vi "SubVi_Flancos.vi"(11 "Alarmas":bool[](array[boolean])) -> (0 "Conteo 3":bool, 1 "Conteo 2":bool, 2 "Conteo 1":bool, 3 "Conteo":bool)   [LabVIEW 2017]
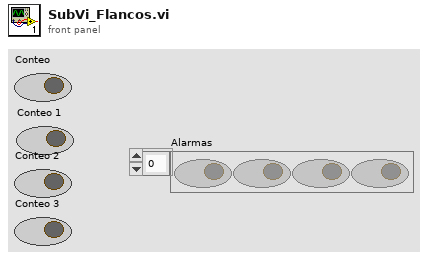
[diagram p1: front panel]
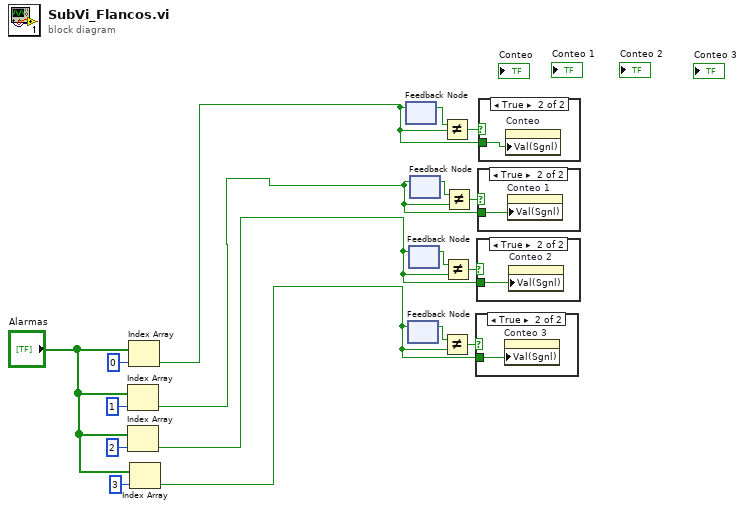
[diagram p0: block diagram]
diagram:
  n1 = Index Array(array="Alarmas", index=1) -> (element=w2:bool)
  n2 = Index Array(array="Alarmas", index=2) -> (element=w3:bool)
  n3 = Index Array(array="Alarmas", index=0) -> (element=w1:bool)
  n4 = Index Array(array="Alarmas", index=3) -> (element=w4:bool)
  n5 = feedback #1() -> (w17:bool)  [unwired: 1 in]
  n6 = feedback-in #1(w1) -> ()
  n7 = feedback #2() -> (w11:bool)  [unwired: 1 in]
  n8 = feedback-in #2(w4) -> ()
  n9 = feedback #3() -> (w13:bool)  [unwired: 1 in]
  n10 = feedback-in #3(w3) -> ()
  n11 = feedback #4() -> (w15:bool)  [unwired: 1 in]
  n12 = feedback-in #4(w2) -> ()
  n13 = Not Equal?(x=w17, y=w1) -> (x != y?=w16:bool)
  n14 = Not Equal?(x=w11, y=w4) -> (x != y?=w10:bool)
  n15 = Not Equal?(x=w13, y=w3) -> (x != y?=w12:bool)
  n16 = Not Equal?(x=w15, y=w2) -> (x != y?=w14:bool)
  n17 = case shown="True" w10 {
    tunnel: w4 -> [_ w18]
    frame False {
    }
    frame True {
      n18 = property on="Conteo 3" class="Bool (strict)"("Val(Sgnl)"=w18) -> ()  [unwired: 2 in, 2 out]
    }
  }
  n19 = case shown="True" w12 {
    tunnel: w3 -> [_ w19]
    frame False {
    }
    frame True {
      n20 = property on="Conteo 2" class="Bool (strict)"("Val(Sgnl)"=w19) -> ()  [unwired: 2 in, 2 out]
    }
  }
  n21 = case shown="True" w14 {
    tunnel: w2 -> [_ w20]
    frame False {
    }
    frame True {
      n22 = property on="Conteo 1" class="Bool (strict)"("Val(Sgnl)"=w20) -> ()  [unwired: 2 in, 2 out]
    }
  }
  n23 = case shown="True" w16 {
    tunnel: w1 -> [_ w21]
    frame False {
    }
    frame True {
      n24 = property on="Conteo" class="Bool (strict)"("Val(Sgnl)"=w21) -> ()  [unwired: 2 in, 2 out]
    }
  }
